vi "Display Single Channel.vi"(8 "Error In":errorcluster, 11 "Waveform Array":waveform(dbl)[][](array[waveform])) -> (0 "Error Out":errorcluster, 1 "Trigger":dynamicdata(graph), 2 "Dev1 Ch3":dynamicdata(graph))   [LabVIEW 2017]
panel:
  out "Dev1":waveform(dbl)[](array[waveform])
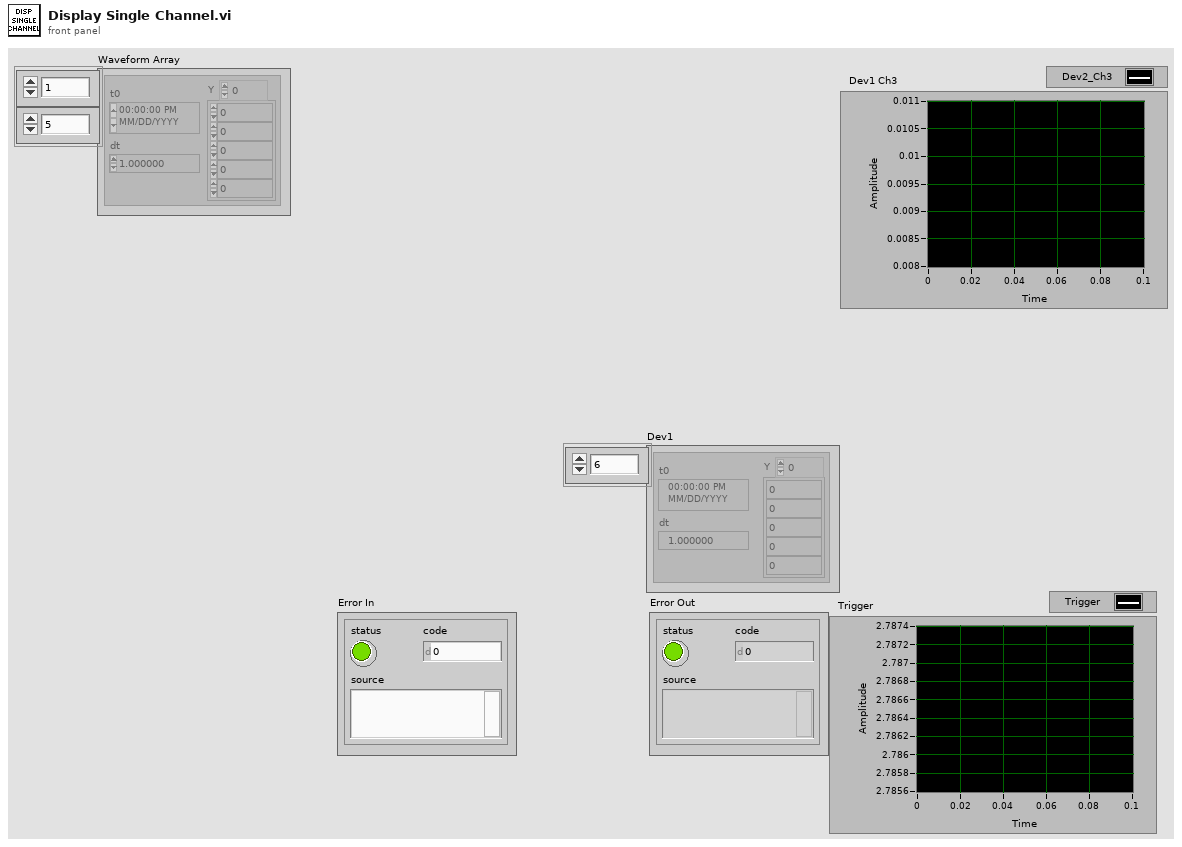
[diagram p1: front panel]
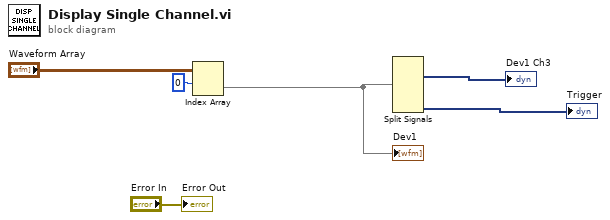
[diagram p0: block diagram]
diagram:
  n1 = Index Array(array="Waveform Array", index (row)=0) -> (element=w3:waveform(dbl)[])  [unwired: 1 in]
  "Dev1" <- w3
  n2 = Split Signals(w3) -> (→"Dev1 Ch3":dynamicdata, →"Trigger":dynamicdata)  [unwired: 7 in, 5 out]
  "Error Out" <- "Error In"
